vi "mandelbrot_2.vi"() -> ()   [LabVIEW 2012]
panel:
  in  "status 2":string="Waiting..."
  in  "Quite":bool
  in  "Z Scale.Marker Values[]":cluster{dbl, u32}[](array[cluster])=[{0.0, 16777222}, {10.0, 16720402}, {20.0, 16776704}, {30.0, 786176}, {40.0, 62719}, {50.0, 4591}, {60.0, 12648703}]
  out "move inc":dbl=0.5
  in  "quality":i32(slide)=800 min=200 max=1000 step=200 scale=200.0..1000.0
  in  "reset":bool
  in  "zoom out":bool
  in  "zoom in":bool
  in  "status":string="Waiting..."
  in  "down":bool
  in  "up":bool
  in  "right":bool
  in  "left":bool
  out "mandelbrot set":ext[][](graph)
  # "zoom"
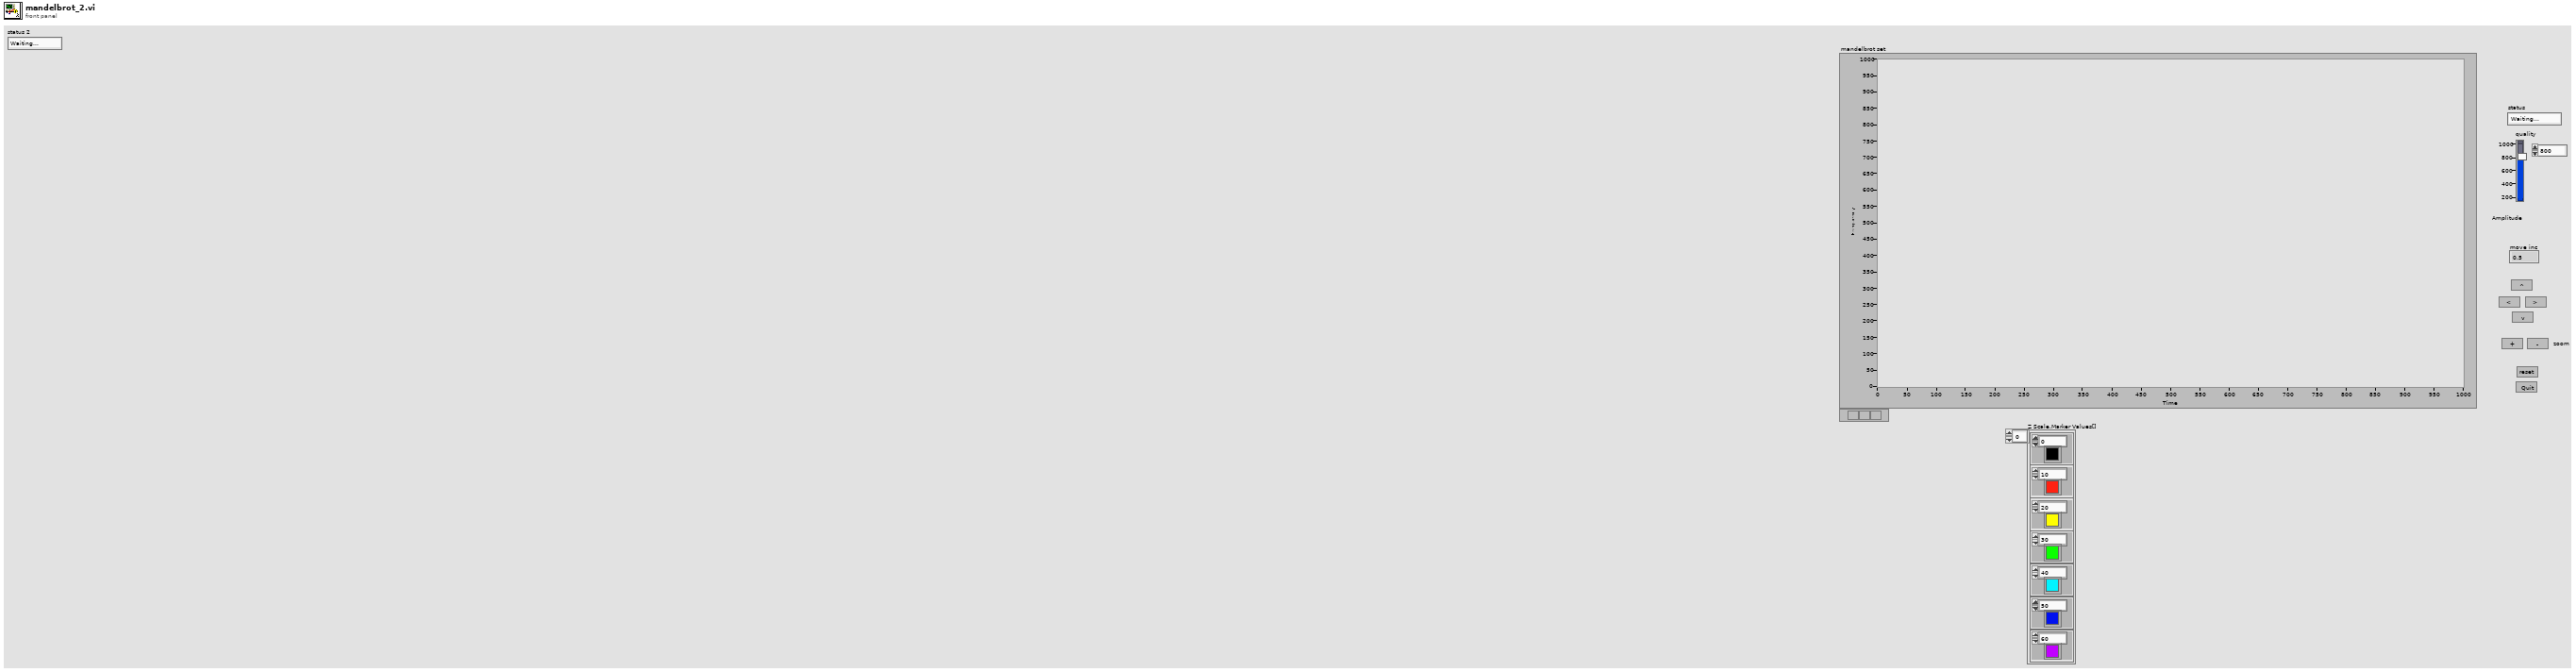
[diagram p1: front panel]
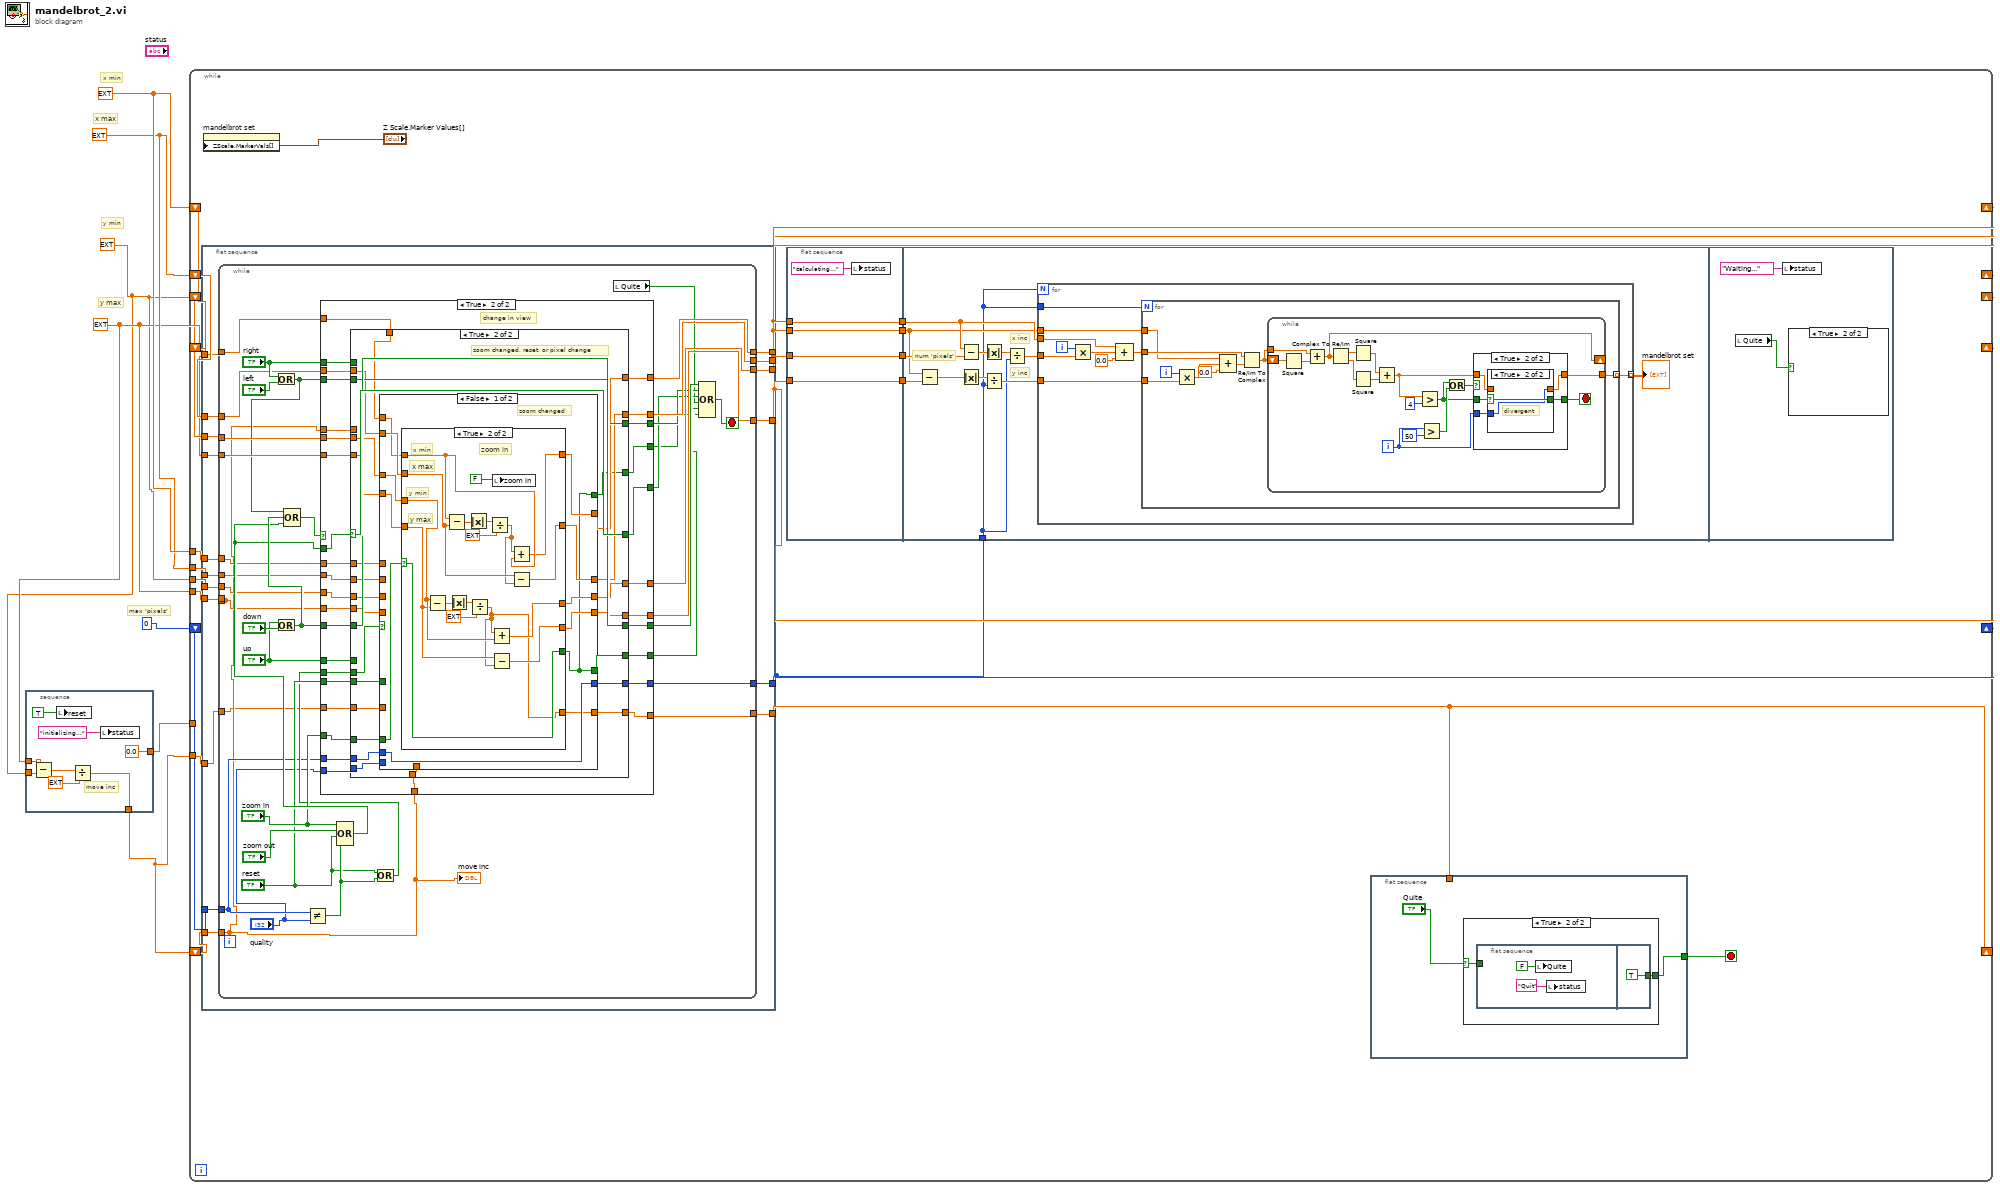
[diagram p0: block diagram]
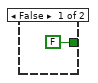
[diagram p2: hidden frame]
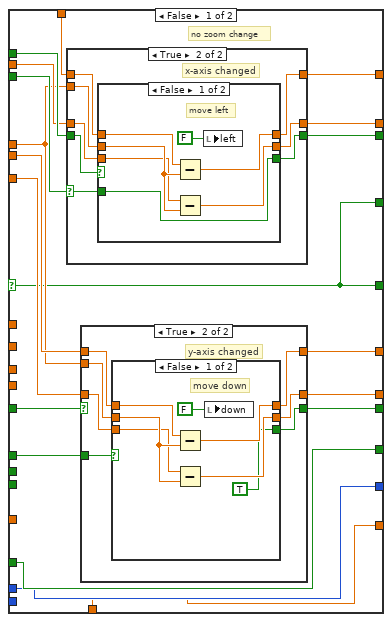
[diagram p4: hidden frame]
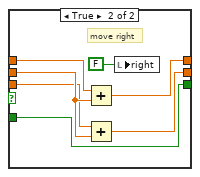
[diagram p6: hidden frame]
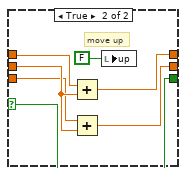
[diagram p8: hidden frame]
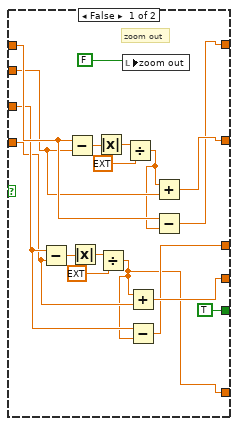
[diagram p9: hidden frame]
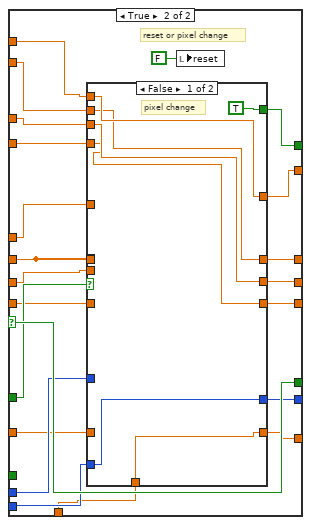
[diagram p10: hidden frame]
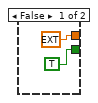
[diagram p13: hidden frame]
diagram:
  w3 = ext 1.0
  w2 = ext -1.0
  w6 = ext 1.0
  w7 = ext -2.0
  # "max 'pixals'"
  # "y max"
  # "y min"
  # "x max"
  # "x min"
  n1 = stacked-sequence {
    tunnel: [0.0 ("Scrollbar")] -> w5
    tunnel: w3 -> [w10]
    tunnel: w2 -> [w9]
    tunnel: [w8] -> w1
    frame #0 {
      # "move inc"
      n2 = Subtract(x=w10, y=w9) -> (x-y=w11:ext)
      n3 = local write "reset"(TRUE ("reset")) -> ()
      n4 = Divide(x=w11, y=ext 4.0) -> (x/y=w8:ext)
      n5 = local write "status"("initializing...") -> ()
    }
  }
  n6 = while {
    shift-right: [w28] -> _
    shift-left: w7 -> [w38]
    shift-right: [w30] -> _
    shift-left: w2 -> [w36]
    shift-right: [w27] -> _
    shift-left: w6 -> [w37]
    shift-right: [w29] -> _
    shift-left: w3 -> [w35]
    tunnel: w7 -> [w26]
    tunnel: w6 -> [w25]
    tunnel: w2 -> [w24]
    tunnel: w3 -> [w23]
    tunnel: w5 -> [_]
    shift-right: [w21] -> _
    shift-left: 0 -> [w22]
    shift-right: [w16] -> _
    shift-left: w1 -> [w20]
    tunnel: w1 -> [w19]
    stop <- w17 stop-if-true
    n7 = flat-sequence {
      tunnel: [w63] -> w29
      tunnel: [w62] -> w30
      tunnel: [w61] -> w28
      tunnel: [w60] -> w27
      tunnel: w38 -> [w59]
      tunnel: w37 -> [w58]
      tunnel: w36 -> [w57]
      tunnel: w35 -> [w56]
      tunnel: w26 -> [w55]
      tunnel: w25 -> [w54]
      tunnel: w24 -> [w53]
      tunnel: w23 -> [w52]
      tunnel: w22 -> [w51]
      tunnel: [w50] -> w21
      tunnel: w20 -> [w49]
      tunnel: [w48] -> w16
      tunnel: w19 -> [w47]
      frame #0 {
        n8 = while {
          tunnel: [w96] -> w63
          tunnel: [w97] -> w62
          tunnel: w56 -> [w101]
          tunnel: w57 -> [w100]
          tunnel: w58 -> [w92]
          tunnel: w59 -> [w93]
          tunnel: [w91] -> w61
          tunnel: [w90] -> w60
          tunnel: w55 -> [w80]
          tunnel: w54 -> [w79]
          tunnel: w53 -> [w78]
          tunnel: [w77] -> _
          tunnel: w52 -> [w77]
          tunnel: w51 -> [w71]
          tunnel: [w69] -> w50
          tunnel: w49 -> [w66]
          tunnel: [w67] -> w48
          tunnel: w47 -> [w65]
          stop <- w87 stop-if-true
          n9 = Or(x="right", y="left") -> (x .or. y?=w86:bool)
          n10 = Or(x="up", y="down") -> (x .or. y?=w85:bool)
          n11 = Not Equal?(x=w71, y="quality") -> (x != y?=w74:bool)
          n12 = Compound Arithmetic op=OR("zoom in", "zoom out", "reset", w74) -> (w81:bool)
          n13 = Compound Arithmetic op=OR(w86, w85, w81) -> (w84:bool)
          n14 = Or(x="reset", y=w74) -> (x .or. y?=w72:bool)
          n15 = case shown="True" w84 {
            selector: w84 -> [w103 _]
            tunnel: w101 -> [w108 w144]
            tunnel: w100 -> [w109 w143]
            tunnel: w85 -> [w107 w142]
            tunnel: "up" -> [w105 w141]
            tunnel: [w109 w140] -> w97
            tunnel: [w108 w139] -> w96
            tunnel: w86 -> [w112 w138]
            tunnel: "right" -> [w106 w137]
            tunnel: w93 -> [w111 w136]
            tunnel: w92 -> [w110 w135]
            tunnel: w66 -> [_ w134]
            tunnel: [w111 w133] -> w91
            tunnel: [w110 w132] -> w90
            tunnel: [w107 w131] -> w89
            tunnel: [w106 w130] -> w88
            tunnel: [w112 w129] -> w83
            tunnel: w81 -> [_ w128]
            tunnel: "reset" -> [_ w127]
            tunnel: w80 -> [_ w126]
            tunnel: w79 -> [_ w125]
            tunnel: w78 -> [_ w124]
            tunnel: w77 -> [_ w123]
            tunnel: [w105 w122] -> w76
            tunnel: "zoom in" -> [_ w121]
            tunnel: w72 -> [_ w120]
            tunnel: w71 -> [w104 w119]
            tunnel: "quality" -> [_ w118]
            tunnel: [w104 w117] -> w69
            tunnel: [w103 w116] -> w68
            tunnel: w66 -> [w102 w115]
            tunnel: [w102 w114] -> w67
            tunnel: w65 -> [_ w113]
            frame False {
              # "no buttons pressed"
            }
            frame True {
              # "change in view"
              n16 = case shown="True" w128 {
                selector: w128 -> [w146 w238]
                tunnel: w144 -> [w163 w226]
                tunnel: w143 -> [w162 w225]
                tunnel: w142 -> [w161 w237]
                tunnel: w141 -> [w160 _]
                tunnel: [w159 w230] -> w140
                tunnel: [w158 w231] -> w139
                tunnel: w138 -> [w157 w236]
                tunnel: w137 -> [w156 _]
                tunnel: w136 -> [w155 w224]
                tunnel: w135 -> [w154 w223]
                tunnel: w134 -> [w153 _]
                tunnel: [w152 w228] -> w133
                tunnel: [w151 w227] -> w132
                tunnel: [w150 w237] -> w131
                tunnel: [w149 w236] -> w130
                tunnel: [w146 w238] -> w129
                tunnel: w127 -> [_ w220]
                tunnel: w126 -> [_ w235]
                tunnel: w125 -> [_ w234]
                tunnel: w124 -> [_ w233]
                tunnel: w123 -> [_ w232]
                tunnel: [w148 w229] -> w122
                tunnel: w121 -> [w148 w222]
                tunnel: w120 -> [_ w221]
                tunnel: w119 -> [w147 w219]
                tunnel: w118 -> [_ w218]
                tunnel: [w147 w217] -> w117
                tunnel: [w146 w216] -> w116
                tunnel: w115 -> [w145 w215]
                tunnel: [w145 w214] -> w114
                tunnel: w113 -> [_ w213]
                frame False {
                  # "no zoom change"
                  n17 = case shown="True" w157 {
                    selector: w157 -> [_ w168]
                    tunnel: w156 -> [w164 w169]
                    tunnel: w155 -> [w166 w174]
                    tunnel: w154 -> [w165 w173]
                    tunnel: w153 -> [_ w172]
                    tunnel: [w166 w171] -> w152
                    tunnel: [w165 w170] -> w151
                    tunnel: [w164 w167] -> w149
                    frame False {
                    }
                    frame True {
                      # "x-axis changed"
                      n18 = case shown="False" w169 {
                        tunnel: [w180 w188] -> w170
                        tunnel: [w181 w187] -> w171
                        tunnel: w172 -> [w179 w186]
                        tunnel: w174 -> [w178 w185]
                        tunnel: w173 -> [w177 w184]
                        tunnel: w168 -> [w175 w182]
                        tunnel: [w175 w182] -> w167
                        frame False {
                          # "move left"
                          n19 = Subtract(x=w178, y=w179) -> (x-y=w181:ext)
                          n20 = Subtract(x=w177, y=w179) -> (x-y=w180:ext)
                          n21 = local write "left"(FALSE ("left")) -> ()
                        }
                        frame True {
                          # "move right"
                          n22 = Add(x=w185, y=w186) -> (x+y=w187:ext)
                          n23 = Add(x=w184, y=w186) -> (x+y=w188:ext)
                          n24 = local write "right"(FALSE ("up")) -> ()
                        }
                      }
                    }
                  }
                  n25 = case shown="True" w161 {
                    tunnel: [w191 w198] -> w159
                    tunnel: w163 -> [w190 w194]
                    tunnel: w162 -> [w191 w195]
                    tunnel: w160 -> [w189 w192]
                    tunnel: [w190 w197] -> w158
                    tunnel: w153 -> [_ w196]
                    tunnel: [w189 w193] -> w150
                    frame False {
                    }
                    frame True {
                      # "y-axis changed"
                      n26 = case shown="False" w192 {
                        selector: w192 -> [_ w206]
                        tunnel: [w204 w211] -> w197
                        tunnel: [w205 w210] -> w198
                        tunnel: w196 -> [w203 w209]
                        tunnel: w195 -> [w202 w208]
                        tunnel: w194 -> [w201 w207]
                        tunnel: [TRUE w206] -> w193
                        frame False {
                          # "move down"
                          n27 = Subtract(x=w202, y=w203) -> (x-y=w205:ext)
                          n28 = Subtract(x=w201, y=w203) -> (x-y=w204:ext)
                          n29 = local write "down"(FALSE ("down")) -> ()
                        }
                        frame True {
                          # "move up"
                          n30 = Add(x=w208, y=w209) -> (x+y=w210:ext)
                          n31 = Add(x=w207, y=w209) -> (x+y=w211:ext)
                          n32 = local write "up"(FALSE ("up")) -> ()
                        }
                      }
                    }
                  }
                }
                frame True {
                  # "zoom changed, reset, or pixel change"
                  n33 = case shown="False" w221 {
                    selector: w221 -> [_ w308]
                    tunnel: w235 -> [_ w305]
                    tunnel: w234 -> [_ w302]
                    tunnel: w233 -> [_ w301]
                    tunnel: w232 -> [_ w299]
                    tunnel: [w245 w304] -> w228
                    tunnel: [w244 w303] -> w227
                    tunnel: [w243 w300] -> w230
                    tunnel: [w242 w298] -> w231
                    tunnel: [w240 w308] -> w229
                    tunnel: w226 -> [w249 w294]
                    tunnel: w225 -> [w248 w295]
                    tunnel: w224 -> [w246 w297]
                    tunnel: w223 -> [w247 w296]
                    tunnel: w222 -> [w250 _]
                    tunnel: w220 -> [_ w306]
                    tunnel: w219 -> [w241 w293]
                    tunnel: w218 -> [_ w292]
                    tunnel: [w241 w291] -> w217
                    tunnel: [w240 w290] -> w216
                    tunnel: w215 -> [_ w287]
                    tunnel: [w239 w288] -> w214
                    tunnel: w213 -> [_ w289]
                    frame False {
                      # "zoom changed"
                      n34 = case shown="True" w250 {
                        selector: w250 -> [_ w274]
                        tunnel: [TRUE w274] -> w240
                        tunnel: w249 -> [w258 w272]
                        tunnel: w248 -> [w259 w273]
                        tunnel: w247 -> [w260 w281]
                        tunnel: w246 -> [w261 w283]
                        tunnel: [w254 w282] -> w245
                        tunnel: [w255 w280] -> w244
                        tunnel: [w256 w276] -> w243
                        tunnel: [w257 w275] -> w242
                        tunnel: [w251 w269] -> w239
                        frame False {
                          # "zoom out"
                          n35 = Subtract(x=w259, y=w258) -> (x-y=w264:ext)
                          n36 = Subtract(x=w261, y=w260) -> (x-y=w267:ext)
                          n37 = Absolute Value(x=w264) -> (abs(x)=w263:ext)
                          n38 = Absolute Value(x=w267) -> (abs(x)=w266:ext)
                          n39 = Divide(x=w263, y=ext 4.0) -> (x/y=w251:ext)
                          n40 = local write "zoom out"(FALSE ("zoom out")) -> ()
                          n41 = Divide(x=w266, y=ext 4.0) -> (x/y=w252:ext)
                          n42 = Add(x=w251, y=w258) -> (x+y=w257:ext)
                          n43 = Subtract(x=w259, y=w251) -> (x-y=w256:ext)
                          n44 = Add(x=w252, y=w260) -> (x+y=w255:ext)
                          n45 = Subtract(x=w261, y=w252) -> (x-y=w254:ext)
                        }
                        frame True {
                          # "y max"
                          # "y min"
                          # "x max"
                          # "x min"
                          # "zoom in"
                          n46 = Subtract(x=w273, y=w272) -> (x-y=w279:ext)
                          n47 = Subtract(x=w283, y=w281) -> (x-y=w285:ext)
                          n48 = Absolute Value(x=w279) -> (abs(x)=w278:ext)
                          n49 = Absolute Value(x=w285) -> (abs(x)=w271:ext)
                          n50 = Divide(x=w278, y=ext 4.0) -> (x/y=w269:ext)
                          n51 = Divide(x=w271, y=ext 4.0) -> (x/y=w270:ext)
                          n52 = Add(x=w269, y=w273) -> (x+y=w276:ext)
                          n53 = Subtract(x=w272, y=w269) -> (x-y=w275:ext)
                          n54 = local write "zoom in"(FALSE ("zoom in")) -> ()
                          n55 = Add(x=w270, y=w283) -> (x+y=w282:ext)
                          n56 = Subtract(x=w281, y=w270) -> (x-y=w280:ext)
                        }
                      }
                    }
                    frame True {
                      # "reset or pixel change"
                      n57 = case shown="False" w306 {
                        selector: w306 -> [_ w317]
                        tunnel: w305 -> [_ w322]
                        tunnel: [w315 w322] -> w304
                        tunnel: [w314 w321] -> w303
                        tunnel: w302 -> [_ _]
                        tunnel: w302 -> [_ w321]
                        tunnel: w301 -> [_ w320]
                        tunnel: [w313 w320] -> w300
                        tunnel: w299 -> [_ w319]
                        tunnel: [w312 w319] -> w298
                        tunnel: w297 -> [w315 _]
                        tunnel: w296 -> [w314 _]
                        tunnel: w295 -> [w313 _]
                        tunnel: w294 -> [w312 _]
                        tunnel: w293 -> [_ w318]
                        tunnel: w292 -> [w311 _]
                        tunnel: [w311 w318] -> w291
                        tunnel: [TRUE w317] -> w290
                        tunnel: w289 -> [_ w316]
                        tunnel: [w309 w316] -> w288
                        tunnel: w287 -> [w309 _]
                        frame False {
                          # "pixel change"
                        }
                        frame True {
                          # "reset"
                        }
                      }
                      n58 = local write "reset"(FALSE ("reset")) -> ()
                    }
                  }
                }
              }
            }
          }
          n59 = local read "Quite"() -> (w64:bool)
          n60 = Compound Arithmetic op=OR(w89, w88, w83, w64, w76, w68) -> (w87:bool)
          "move inc" <- w66
        }
      }
    }
    n61 = property on="mandelbrot set" class="IntGraph (strict)"("ZScale.MarkerVals[]"="Z Scale.Marker Values[]") -> ()  [unwired: 2 in, 2 out]
    n62 = flat-sequence {
      tunnel: [w324] -> w34
      tunnel: [w325] -> w33
      tunnel: [w326] -> w32
      tunnel: [w323] -> w31
      tunnel: w30 -> [w323]
      tunnel: w29 -> [w326]
      tunnel: w28 -> [w325]
      tunnel: w27 -> [w324]
      tunnel: w34 -> [w330]
      tunnel: w33 -> [w331]
      tunnel: w32 -> [w332]
      tunnel: w31 -> [w329]
      tunnel: w21 -> [w328]
      frame #0 {
        n63 = local write "status"("calculating...") -> ()
      }
      frame #1 {
        # "y inc"
        # "x inc"
        # "num 'pixels'"
        n64 = Subtract(x=w329, y=w332) -> (x-y=w337:ext)
        n65 = Subtract(x=w331, y=w330) -> (x-y=w339:ext)
        n66 = Absolute Value(x=w337) -> (abs(x)=w336:ext)
        n67 = Absolute Value(x=w339) -> (abs(x)=w338:ext)
        n68 = Divide(x=w336, y=w328) -> (x/y=w334:ext)
        n69 = Divide(x=w338, y=w328) -> (x/y=w335:ext)
        n70 = for {
          N: w328 -> [_]
          tunnel: w335 -> [w348]
          tunnel: w334 -> [w347]
          tunnel: w328 -> [w346]
          tunnel: [w342] -> w333 mode=indexing
          tunnel: w331 -> [w341]
          tunnel: w329 -> [w340]
          i -> [w349]
          n71 = Multiply(x=w349, y=w348) -> (x*y=w344:dbl)
          n72 = Compound Arithmetic op=unknown(w341, w344, 0.0 ("y")) -> (w345:ext)
          n73 = for {
            N: w346 -> [_]
            tunnel: w347 -> [w357]
            tunnel: w345 -> [w356]
            tunnel: [w351] -> w342 mode=indexing
            tunnel: w340 -> [w350]
            i -> [w358]
            n74 = Multiply(x=w358, y=w357) -> (x*y=w354:dbl)
            n75 = Compound Arithmetic op=unknown(w350, w354, 0.0 ("y")) -> (w353:ext)
            n76 = Re/Im To Complex(1:w353, 2:w356) -> (0:w352:cxt)
            n77 = while {
              shift-right: [w366] -> _
              shift-left: w352 -> [w368]
              tunnel: w352 -> [w367]
              tunnel: [w361] -> w351
              i -> [w360]
              stop <- w359 stop-if-true
              n78 = Square(x=w368) -> (x^2=w370:cxt)
              n79 = Add(x=w367, y=w370) -> (x+y=w366:cxt)
              n80 = Complex To Re/Im(x + iy=w366) -> (x=w374:ext, y=w375:ext)
              n81 = Square(x=w374) -> (x^2=w373:ext)
              n82 = Square(x=w375) -> (x^2=w372:ext)
              n83 = Add(x=w373, y=w372) -> (x+y=w369:ext)
              n84 = Greater?(x=w369, y=4) -> (0:w362:bool)
              n85 = Greater?(x=w360, y=50) -> (0:w364:bool)
              n86 = Or(x=w362, y=w364) -> (x .or. y?=w363:bool)
              n87 = case shown="True" w363 {
                selector: w363 -> [w377 _]
                tunnel: [w376 w379] -> w361
                tunnel: w369 -> [w376 w382]
                tunnel: [w377 w380] -> w359
                tunnel: w362 -> [_ w381]
                tunnel: w360 -> [_ w378]
                frame False {
                }
                frame True {
                  n88 = case shown="True" w381 {
                    selector: w381 -> [_ w386]
                    tunnel: [ext 0.0 w385] -> w379
                    tunnel: w382 -> [_ _]
                    tunnel: [TRUE w386] -> w380
                    tunnel: w378 -> [_ w385]
                    frame False {
                    }
                    frame True {
                      # "divergent"
                    }
                  }
                }
              }
            }
          }
        }
        "mandelbrot set" <- w333
      }
      frame #2 {
        n89 = local read "Quite"() -> (w387:bool)
        n90 = local write "status"("Waiting...") -> ()
        n91 = case shown="True" w387 {
          frame False {
          }
          frame True {
            n92 = local write "status 2"("Waiting...") -> ()
          }
        }
      }
    }
    n93 = flat-sequence {
      tunnel: [w39] -> w17
      tunnel: w16 -> [_]
      frame #0 {
        n94 = case shown="True" "Quite" {
          selector: "Quite" -> [_ w43]
          tunnel: [FALSE w42] -> w39
          frame False {
          }
          frame True {
            n95 = flat-sequence {
              tunnel: w43 -> [_]
              tunnel: [TRUE] -> w42
              frame #0 {
                n96 = local write "Quite"(FALSE ("stop")) -> ()
                n97 = local write "status"("Quit" ("status")) -> ()
              }
              frame #1 {
              }
            }
          }
        }
      }
    }
  }
